vi "SetDefaults.vi"(8 "error in (no error)":errorcluster, 11 "Service Details In":T1) -> (0 "error out":errorcluster, 2 "Service":T2, 3 "Service Details Out":T1)   [LabVIEW 2019, in "MicronClient.lvclass"]
uses:
  MicronClient.lvclass
  MicronCLI/Typedefs/ServiceDetails.ctl
  Typedefs/ServiceDetails.ctl
  MicronCLI/MicronCLI.lvclass
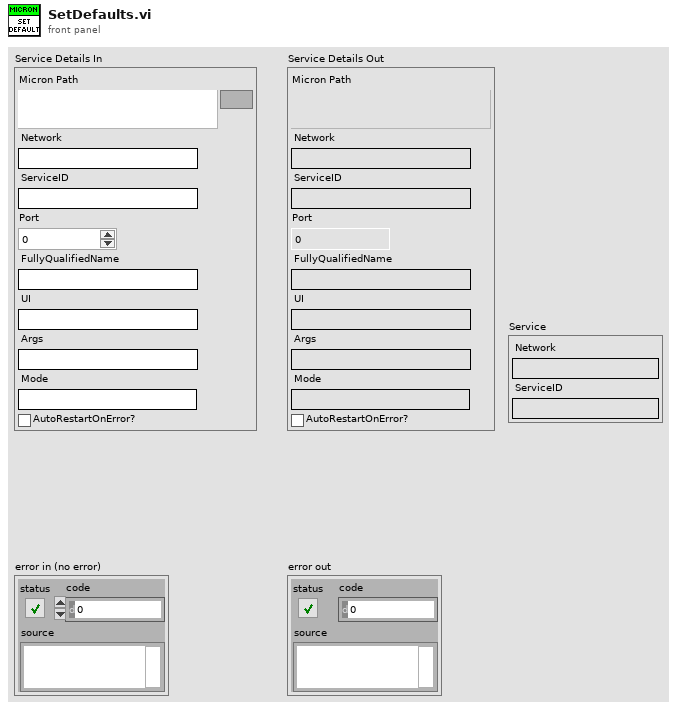
[diagram p1: front panel]
types:
  T1 = typedef "MicronClient.lvclass/ServiceDetails.ctl" = cluster{"Micron Path":path, "Network":string, "ServiceID":string, "Port":i32, "FullyQualifiedName":string, "UI":string, "Args":string, "Mode":string, "AutoRestartOnError?":bool}
  T2 = typedef "MicronCLI.lvclass/ServiceDetails.ctl" = cluster{"Network":string, "ServiceID":string}
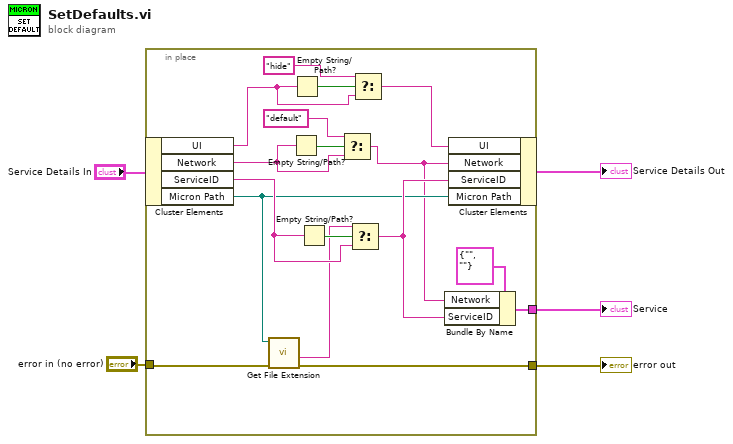
[diagram p0: block diagram]
diagram:
  n1 = in-place {
    in-place-border: "error in (no error)" -> [w19]
    in-place-border: [w15] -> w3
    in-place-border: [w6] -> w5
    n2 = in-place-cluster #1("Service Details In") -> ("UI"=w11:string, "Network"=w21:string, "ServiceID"=w17:string, "Micron Path"=w14:path)
    n3 = call <vilib>:"Get File Extension.vi"("error in (no error)"=w19, "file"=w14) -> ("error out"=w15:errorcluster, "filename without extension"=w13:string)  [unwired: 5 in, 3 out]
    n4 = Empty String/Path?(string/path=w21) -> (empty?=w22:bool)
    n5 = Empty String/Path?(string/path=w11) -> (empty?=w12:bool)
    n6 = Empty String/Path?(string/path=w17) -> (empty?=w18:bool)
    n7 = Select(t="default", s=w22, f=w21) -> (s? t:f=w8:string)
    n8 = Select(t=w13, s=w18, f=w17) -> (s? t:f=w16:string)
    n9 = Select(t="hide", s=w12, f=w11) -> (s? t:f=w9:string)
    n10 = Bundle By Name(cluster=T2 {"Network"="", "ServiceID"=""} ("Service"), "Network"=w8, "ServiceID"=w16) -> (w6:T2)
    n11 = in-place-cluster #1("UI"=w9, "Network"=w8, "ServiceID"=w16, "Micron Path"=w14) -> (→"Service Details Out":T1)
  }
  "Service" <- w5
  "error out" <- w3
